vi "Simple_Communication.vi"() -> ()   [LabVIEW 2023]
uses:
  LabVIEW/Lab4_235/Serial - Settings.ctl
  <vilib>/Instr/_visa.llb/VISA Configure Serial Port (Instr).vi
panel:
  in  "write buffer":string
  in  "stop":bool
  out "read buffer":string
  in  "Serial Settings":T1={"baud rate"=115200, "data bits"=8, "parity"=enum."None", "stop bits"=10, "flow control"=0} {"flow control" items=["None"=0, "XON/XOFF"=1, "RTS/CTS"=2, "DTR/DSR"=4]; "stop bits" items=["1.0"=10, "1.5"=15, "2.0"=20]; "data bits" min=5 max=8 step=1; "baud rate" items=["75"=75, "110"=110, "134"=134, "150"=150, "300"=300, "600"=600, "1200"=1200, "1800"=1800, "2400"=2400, "4800"=4800, "7200"=7200, "9600"=9600, "14400"=14400, "19200"=19200, "28800"=28800, "38400"=38400, "56000"=56000, "57600"=57600, "115200"=115200, "128000"=128000, "230400"=230400]}
  in  "VISA resource name":refnum<visa-resource-name>
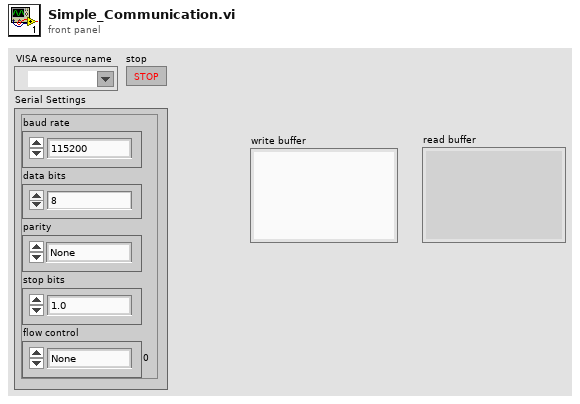
[diagram p1: front panel]
types:
  T1 = typedef "Serial - Settings.ctl" = cluster{"baud rate":u32, "data bits":u16, "parity":enum16{"None", "Odd", "Even", "Mark", "Space"}, "stop bits":u16, "flow control":u16}
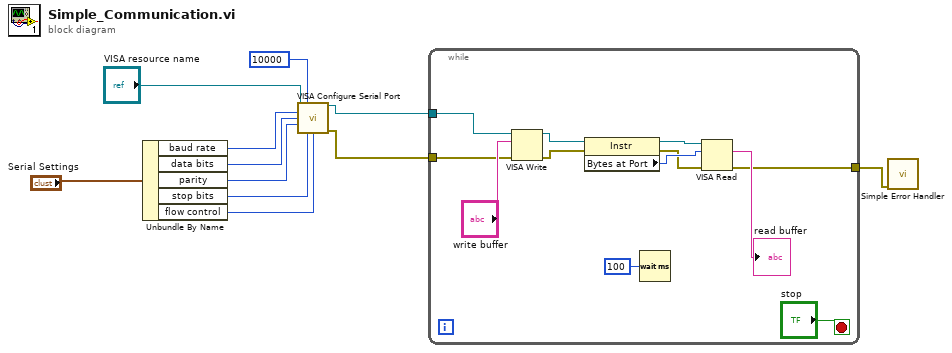
[diagram p0: block diagram]
diagram:
  n1 = Unbundle By Name("Serial Settings") -> ("baud rate"=w9:u32, "data bits"=w8:u16, "parity"=w7:enum16{"None", "Odd", "Even", "Mark", "Space"}, "stop bits"=w6:u16, "flow control"=w5:u16)
  n2 = call-poly "VISA Configure Serial Port"("VISA resource name"="VISA resource name", "timeout (10sec)"=u32 10000, "baud rate (9600)"=w9, "data bits (8)"=w8, "parity (0:none)"=w7, "stop bits (10: 1 bit)"=w6, "flow control (0:none)"=w5) -> ("VISA resource name out"=w3:refnum<visa-resource-name>, "error out"=w2:errorcluster)  [unwired: 7 in]
  n3 = while {
    tunnel: w3 -> [w18]
    tunnel: w2 -> [w16]
    tunnel: [w13] -> w1
    stop <- "stop" stop-if-true
    n4 = VISA Write(VISA resource name=w18, write buffer="write buffer", error in (no error)=w16) -> (VISA resource name out=w21:refnum<visa-resource-name>, error out=w15:errorcluster)  [unwired: 1 out]
    n5 = property on="Property Node" class="Instr"(reference=w21, error in=w15) -> (reference out=w22:refnum<visa-resource-name>, error out=w14:errorcluster, "Bytes at Port"=w23:u32)
    n6 = Wait (ms)(milliseconds to wait=u32 100) -> ()  [unwired: 1 out]
    n7 = VISA Read(VISA resource name=w22, byte count=w23, error in (no error)=w14) -> (read buffer=→"read buffer":string, error out=w13:errorcluster)  [unwired: 2 out]
  }
  n8 = call <vilib>:"Simple Error Handler.vi"("error in (no error)"=w1) -> ()  [unwired: 4 in, 5 out]
